vi "手机号码显示.vi"(11 "手机号码内容":u8[](array[numeric])) -> (3 "字符串":string)   [LabVIEW 2015]
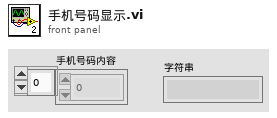
[diagram p1: front panel]
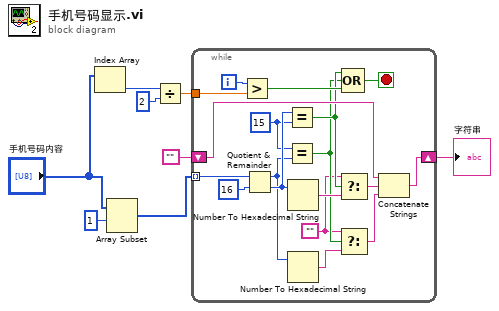
[diagram p0: block diagram]
diagram:
  n1 = Index Array(array="手机号码内容") -> (element=w4:u8)  [unwired: 1 in]
  n2 = Array Subset(array="手机号码内容", index=1 ("索引")) -> (w2:u8[])  [unwired: 1 in]
  n3 = Divide(x=w4, y=u8 2) -> (x/y=w8:dbl)
  n4 = while {
    tunnel: w2 -> [w26] mode=indexing
    shift-right: [w23] -> w7
    shift-left: "" -> [w24]
    tunnel: w8 -> [w10]
    i -> [w9]
    stop <- w19 stop-if-true
    w11 = ""
    w21 = u8 15 ("y")
    n5 = Greater?(x=w9, y=w10) -> (0:w18:bool)
    n6 = Quotient & Remainder(x=w26, y=u8 16) -> (x-y*floor(x/y)=w20:u8, floor(x/y)=w22:u8)
    n7 = Equal?(x=w22, y=w21) -> (x = y?=w17:bool)
    n8 = Equal?(x=w21, y=w20) -> (x = y?=w12:bool)
    n9 = Number To Hexadecimal String(2:w22) -> (0:w15:string)  [unwired: 1 in]
    n10 = Number To Hexadecimal String(2:w20) -> (0:w13:string)  [unwired: 1 in]
    n11 = Select(t=w11, s=w17, f=w15) -> (s? t:f=w16:string)
    n12 = Select(t=w11, s=w12, f=w13) -> (s? t:f=w14:string)
    n13 = Compound Arithmetic op=OR ("复合运算")(w17, w12, w18) -> (w19:bool)
    n14 = Concatenate Strings(w24, w16, w14) -> (w23:string)
  }
  "字符串" <- w7
